vi "timer.vi"() -> ()   [LabVIEW 2014]
panel:
  in  "start":bool
  in  "stop":bool
  out "time":string
  out "negative":bool
  in  "ss":dbl
  in  "mm":dbl
  in  "hh":dbl
  # "PS:run後要記得按start才會開始跑"
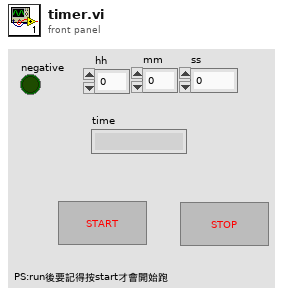
[diagram p1: front panel]
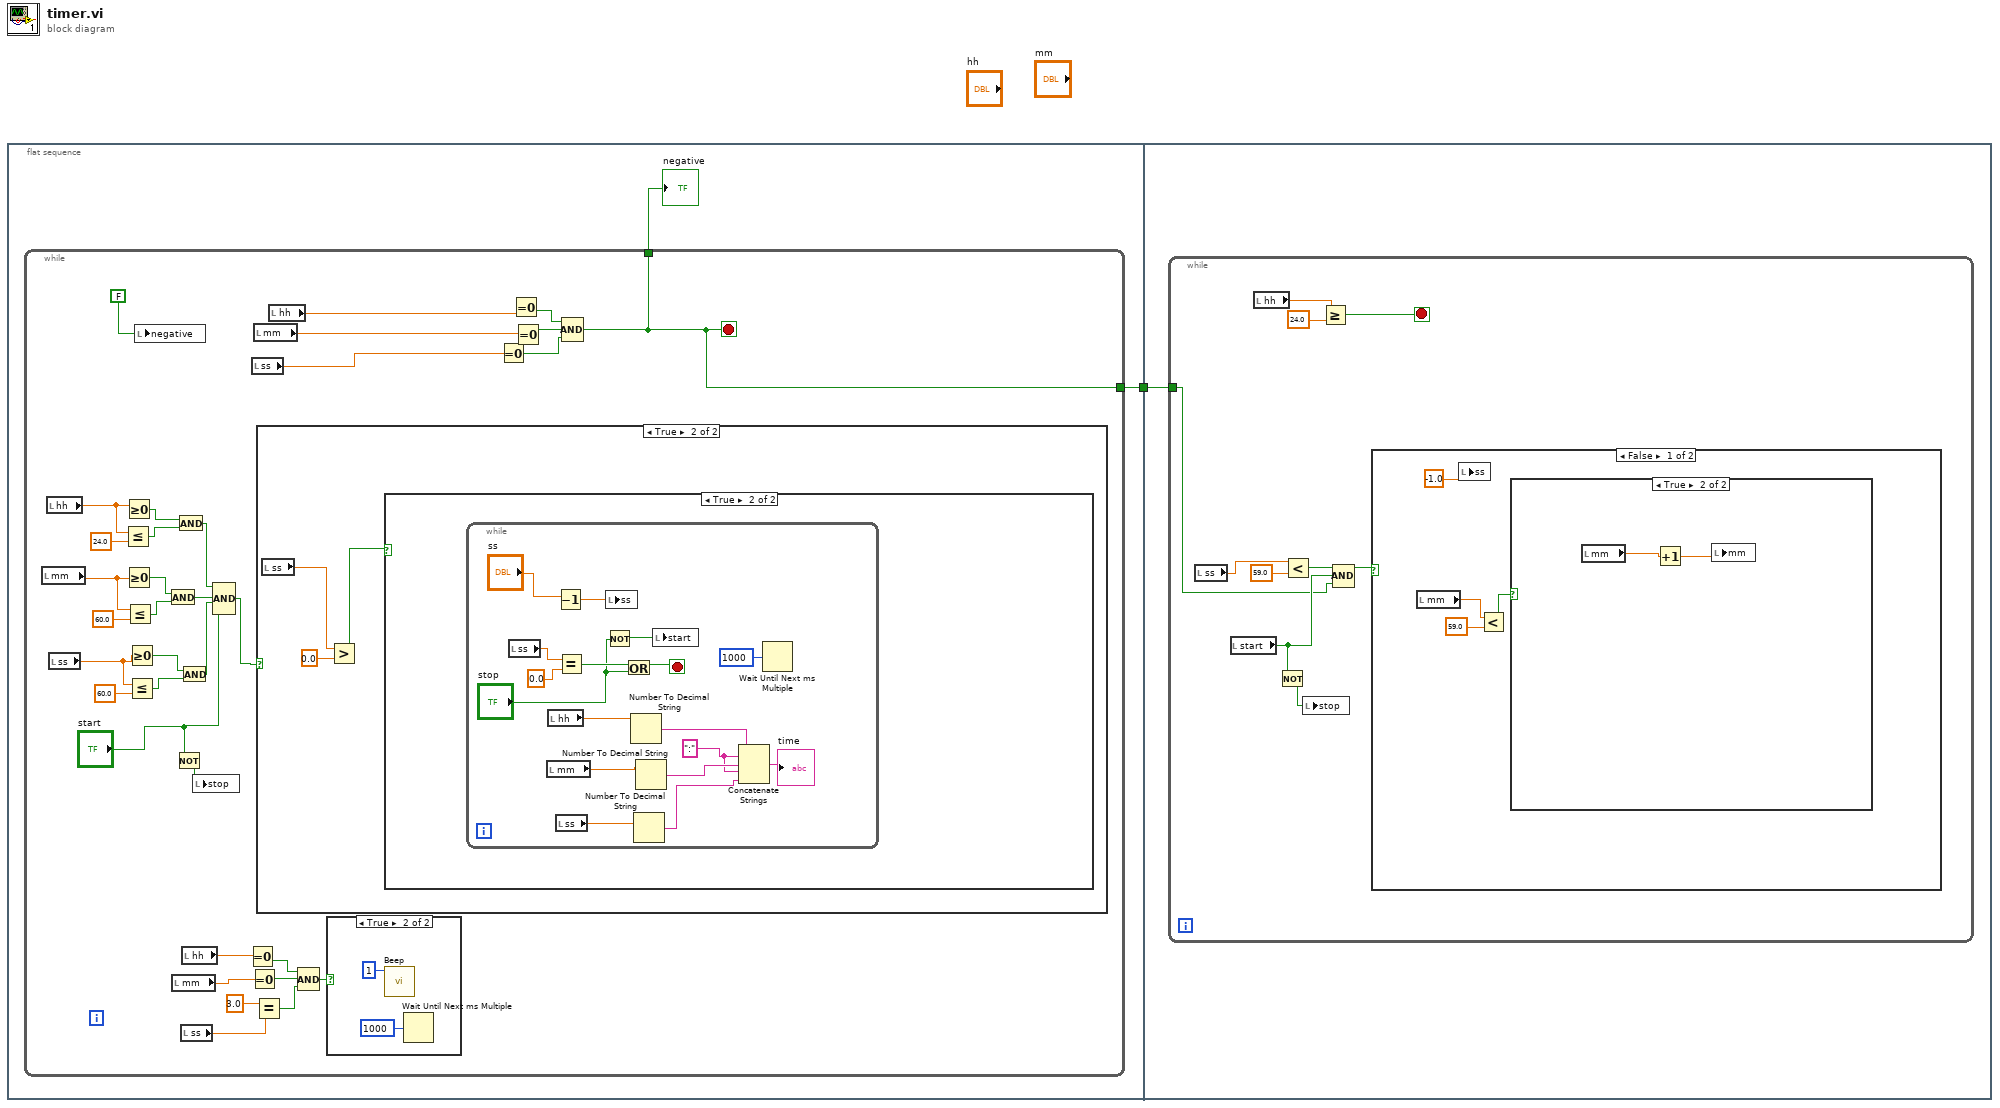
[diagram p0: block diagram]
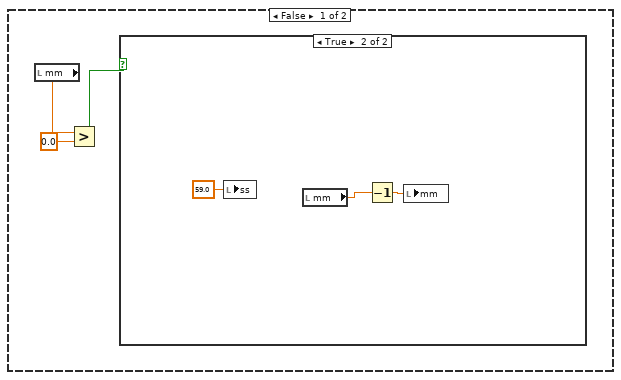
[diagram p4: hidden frame]
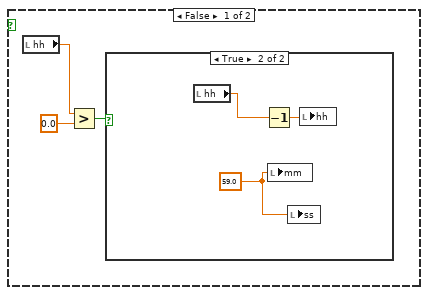
[diagram p5: hidden frame]
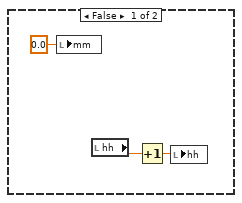
[diagram p7: hidden frame]
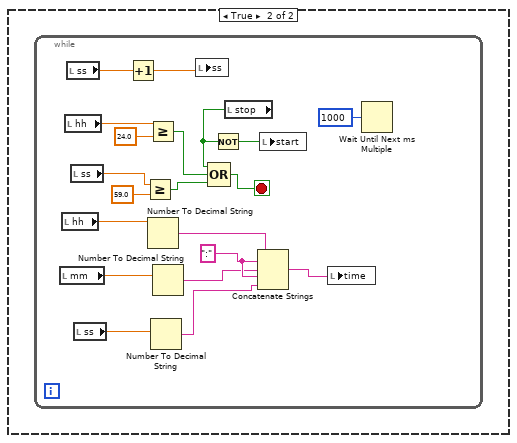
[diagram p8: hidden frame]
diagram:
  n1 = flat-sequence {
    tunnel: [w2] -> w1
    tunnel: w1 -> [w72]
    frame #0 {
      n2 = while {
        tunnel: [w4] -> w3
        tunnel: [w4] -> w2
        stop <- w4 stop-if-true
        n3 = local read "mm"() -> (w17:dbl)
        n4 = local read "hh"() -> (w16:dbl)
        n5 = local read "ss"() -> (w15:dbl)
        n6 = Less Or Equal?(x=w16, y=24.0) -> (x <= y?=w28:bool)
        n7 = Greater Or Equal To 0?(x=w16) -> (x >= 0?=w29:bool)
        n8 = Greater Or Equal To 0?(x=w17) -> (x >= 0?=w27:bool)
        n9 = Less Or Equal?(x=w17, y=60.0) -> (x <= y?=w26:bool)
        n10 = Greater Or Equal To 0?(x=w15) -> (x >= 0?=w25:bool)
        n11 = Less Or Equal?(x=w15, y=60.0) -> (x <= y?=w24:bool)
        n12 = local write "negative"(FALSE ("negative")) -> ()
        n13 = And(x=w27, y=w26) -> (x .and. y?=w22:bool)
        n14 = local read "mm"() -> (w11:dbl)
        n15 = Not(x="start") -> (.not. x?=w6:bool)
        n16 = And(x=w29, y=w28) -> (x .and. y?=w23:bool)
        n17 = And(x=w25, y=w24) -> (x .and. y?=w21:bool)
        n18 = local read "ss"() -> (w12:dbl)
        n19 = local read "hh"() -> (w10:dbl)
        n20 = local write "stop"(w6) -> ()
        n21 = Compound Arithmetic op=AND(w23, w22, w21, "start") -> (w18:bool)
        n22 = Equal To 0?(x=w10) -> (x = 0?=w8:bool)
        n23 = Equal To 0?(x=w11) -> (x = 0?=w7:bool)
        n24 = local read "ss"() -> (w32:dbl)
        n25 = local read "mm"() -> (w33:dbl)
        n26 = Equal?(x=3.0, y=w12) -> (x = y?=w9:bool)
        n27 = case shown="True" w18 {
          frame False {
          }
          frame True {
            n28 = local read "ss"() -> (w41:dbl)
            n29 = Greater?(x=w41, y=0.0) -> (0:w42:bool)
            n30 = case shown="True" w42 {
              frame False {
                n31 = local read "mm"() -> (w44:dbl)
                n32 = Greater?(x=w44, y=0.0) -> (0:w45:bool)
                n33 = case shown="True" w45 {
                  frame False {
                    n34 = local read "hh"() -> (w47:dbl)
                    n35 = Greater?(x=w47, y=0.0) -> (0:w48:bool)
                    n36 = case shown="True" w48 {
                      frame False {
                      }
                      frame True {
                        w49 = 59.0 ("mm")
                        n37 = local read "hh"() -> (w50:dbl)
                        n38 = Decrement(x=w50) -> (x-1=w51:dbl)
                        n39 = local write "mm"(w49) -> ()
                        n40 = local write "ss"(w49) -> ()
                        n41 = local write "hh"(w51) -> ()
                      }
                    }
                  }
                  frame True {
                    n42 = local write "ss"(59.0 ("ss")) -> ()
                    n43 = local read "mm"() -> (w52:dbl)
                    n44 = Decrement(x=w52) -> (x-1=w53:dbl)
                    n45 = local write "mm"(w53) -> ()
                  }
                }
              }
              frame True {
                n46 = while {
                  stop <- w57 stop-if-true
                  w60 = ":" ("string")
                  n47 = local read "ss"() -> (w69:dbl)
                  n48 = local read "mm"() -> (w65:dbl)
                  n49 = local read "hh"() -> (w64:dbl)
                  n50 = Decrement(x="ss") -> (x-1=w68:dbl)
                  n51 = local read "ss"() -> (w66:dbl)
                  n52 = Equal?(x=w69, y=0.0) -> (x = y?=w67:bool)
                  n53 = Not(x="stop") -> (.not. x?=w56:bool)
                  n54 = local write "ss"(w68) -> ()
                  n55 = Or(x=w67, y="stop") -> (x .or. y?=w57:bool)
                  n56 = Number To Decimal String(number=w64) -> (decimal integer string=w63:string)  [unwired: 1 in]
                  n57 = Number To Decimal String(number=w66) -> (decimal integer string=w61:string)  [unwired: 1 in]
                  n58 = Number To Decimal String(number=w65) -> (decimal integer string=w62:string)  [unwired: 1 in]
                  n59 = local write "start"(w56) -> ()
                  n60 = Concatenate Strings(w63, w60, w62, w60, w61) -> (→"time":string)
                  n61 = Wait Until Next ms Multiple(millisecond multiple=u32 1000) -> ()  [unwired: 1 out]
                }
              }
            }
          }
        }
        n62 = local read "hh"() -> (w34:dbl)
        n63 = Compound Arithmetic op=AND(w8, w7, w9) -> (w14:bool)
        n64 = case shown="True" w14 {
          frame False {
          }
          frame True {
            n65 = call <vilib>:"Beep.vi"("frequency (Hz)"=u32 1) -> ()  [unwired: 11 in]
            n66 = Wait Until Next ms Multiple(millisecond multiple=u32 1000) -> ()  [unwired: 1 out]
          }
        }
        n67 = Equal To 0?(x=w32) -> (x = 0?=w35:bool)
        n68 = Equal To 0?(x=w34) -> (x = 0?=w36:bool)
        n69 = Equal To 0?(x=w33) -> (x = 0?=w37:bool)
        n70 = Compound Arithmetic op=AND(w36, w37, w35) -> (w4:bool)
      }
      "negative" <- w3
    }
    frame #1 {
      n71 = while {
        tunnel: w72 -> [w73]
        stop <- w81 stop-if-true
        n72 = local read "ss"() -> (w78:dbl)
        n73 = local read "start"() -> (w75:bool)
        n74 = local read "hh"() -> (w82:dbl)
        n75 = Not(x=w75) -> (.not. x?=w74:bool)
        n76 = Less?(x=w78, y=59.0) -> (x < y?=w79:bool)
        n77 = local write "stop"(w74) -> ()
        n78 = Greater Or Equal?(x=w82, y=24.0) -> (x >= y?=w81:bool)
        n79 = Compound Arithmetic op=AND(w79, w75, w73) -> (w76:bool)
        n80 = case shown="False" w76 {
          frame False {
            n81 = local read "mm"() -> (w84:dbl)
            n82 = local write "ss"(-1.0 ("y")) -> ()
            n83 = Less?(x=w84, y=59.0) -> (x < y?=w85:bool)
            n84 = case shown="True" w85 {
              frame False {
                n85 = local write "mm"(0.0 ("mm")) -> ()
                n86 = local read "hh"() -> (w88:dbl)
                n87 = Increment(x=w88) -> (x+1=w87:dbl)
                n88 = local write "hh"(w87) -> ()
              }
              frame True {
                n89 = local read "mm"() -> (w91:dbl)
                n90 = Increment(x=w91) -> (x+1=w90:dbl)
                n91 = local write "mm"(w90) -> ()
              }
            }
          }
          frame True {
            n92 = while {
              stop <- w96 stop-if-true
              w102 = ":" ("string")
              n93 = local read "mm"() -> (w104:dbl)
              n94 = local read "hh"() -> (w103:dbl)
              n95 = local read "hh"() -> (w98:dbl)
              n96 = local read "ss"() -> (w111:dbl)
              n97 = local read "ss"() -> (w108:dbl)
              n98 = local read "ss"() -> (w105:dbl)
              n99 = Increment(x=w111) -> (x+1=w110:dbl)
              n100 = Greater Or Equal?(x=w108, y=59.0) -> (x >= y?=w94:bool)
              n101 = Greater Or Equal?(x=w98, y=24.0) -> (x >= y?=w95:bool)
              n102 = Number To Decimal String(number=w103) -> (decimal integer string=w99:string)  [unwired: 1 in]
              n103 = Number To Decimal String(number=w105) -> (decimal integer string=w101:string)  [unwired: 1 in]
              n104 = Number To Decimal String(number=w104) -> (decimal integer string=w100:string)  [unwired: 1 in]
              n105 = local write "ss"(w110) -> ()
              n106 = local read "stop"() -> (w93:bool)
              n107 = Compound Arithmetic op=OR(w93, w95, w94) -> (w96:bool)
              n108 = Not(x=w93) -> (.not. x?=w92:bool)
              n109 = Concatenate Strings(w99, w102, w100, w102, w101) -> (w106:string)
              n110 = local write "start"(w92) -> ()
              n111 = local write "time"(w106) -> ()
              n112 = Wait Until Next ms Multiple(millisecond multiple=u32 1000) -> ()  [unwired: 1 out]
            }
          }
        }
      }
    }
  }
